vi "ep_Frequency Time Aggregation.vi"(0 "frequency (1/2) (half cycle)":dbl, 1 "restart (F)":bool, 5 "aggregation settings":T1={"interval"=1, "interval unit"=enum."Runs", "synchronization of intervals"=enum."Not synchronized", "algorithm"=enum."Average"}, 7 "voltage flags":bool[](array[boolean]), 9 "data time stamp":timestamp, 11 "error in (no error)":errorcluster) -> (6 "aggregated frequency":dbl, 8 "aggregated voltage flags":bool[](array[boolean]), 13 "aggregated data time stamp":timestamp, 14 "aggregated data valid?":bool, 15 "error out":errorcluster)   [LabVIEW 2011, in "NI_EP_Power Quality.lvlib"]
doc: "This VI accumulates input data. At every end of specified aggregation interval a minimum value, maximum value and average or RMS found within aggregation interval are provided on output. After this, the accumulation buffers are cleared and accumulation is automatically restarted."
uses:
  <vilib>/addons/Electrical Power/PQ/NI_EP_Power Quality.lvlib
  <vilib>/addons/Electrical Power/PQ/Common/Controls/ep_Aggregation Settings.ctl
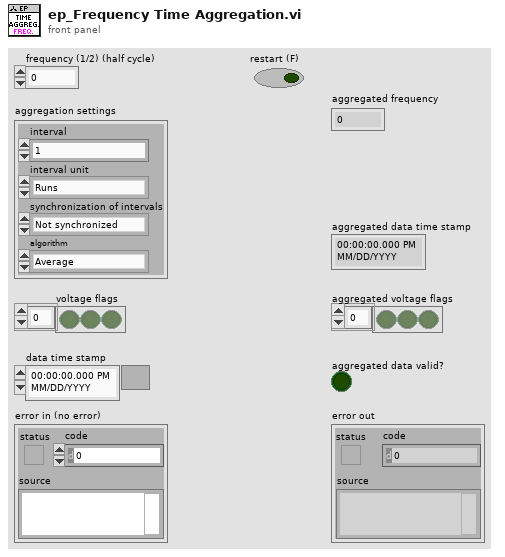
[diagram p1: front panel]
types:
  T1 = typedef "NI_EP_Power Quality.lvlib/ep_Aggregation Settings.ctl" = cluster{"interval":u32, "interval unit":enum16{"Runs", "Seconds", "Minutes", "Hours", "Days", "Weeks"}, "synchronization of intervals":enum16{"Not synchronized", "Interval rounded"}, "algorithm":enum16{"Average", "RMS"}}
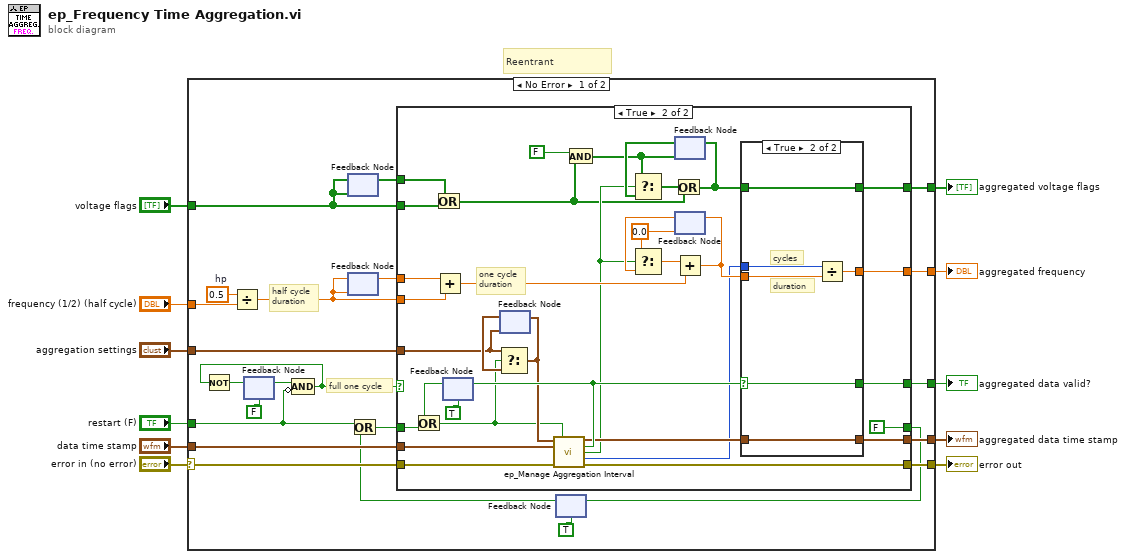
[diagram p0: block diagram]
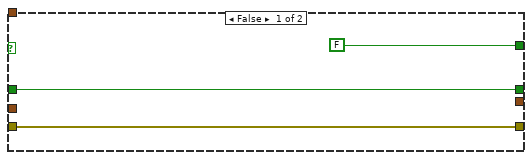
[diagram p2: hidden frame]
diagram:
  # "Reentrant"
  n1 = case shown="No Error" "error in (no error)" {
    selector: "error in (no error)" -> [w30 w79]
    tunnel: "restart (F)" -> [w19 _]
    tunnel: "frequency (1/2) (half cycle)" -> [w16 _]
    tunnel: "aggregation settings" -> [w28 _]
    tunnel: "data time stamp" -> [w34 _]
    tunnel: [w33 w79] -> w8
    tunnel: [w29 _] -> w7
    tunnel: [w32 _] -> w6
    tunnel: [w31 _] -> w5
    tunnel: "voltage flags" -> [w13 _]
    tunnel: [w14 _] -> w1
    frame No Error {
      w17 = 0.5  # hp
      # "half cycle\nduration"
      # "full one cycle"
      n2 = Divide(x=w17, y=w16) -> (x/y=w15:dbl)
      n3 = feedback #1(FALSE) -> (w27:bool)
      n4 = Compound Arithmetic op=AND(w27, invert w19) -> (w24:bool)
      n5 = Not(x=w24) -> (.not. x?=w26:bool)
      n6 = feedback-in #1(w26) -> ()
      n7 = feedback-in #2(w13) -> ()
      n8 = feedback #2(w13) -> (w12:bool[])
      n9 = feedback-in #3(w15) -> ()
      n10 = feedback #3(w15) -> (w23:dbl)
      n11 = feedback #4(TRUE) -> (w20:bool)
      n12 = Or(x=w19, y=w20) -> (x .or. y?=w18:bool)
      n13 = case shown="True" w24 {
        tunnel: w34 -> [_ w67]
        tunnel: [w36 w66] -> w33
        tunnel: [_ w64] -> w32
        tunnel: [_ w62] -> w31
        tunnel: w30 -> [w36 w61]
        tunnel: [FALSE w60] -> w29
        tunnel: w28 -> [_ w58]
        tunnel: w15 -> [_ w49]
        tunnel: w18 -> [w35 w53]
        tunnel: w23 -> [_ w50]
        tunnel: [w35 FALSE ("restart (F)")] -> w21
        tunnel: w13 -> [_ w39]
        tunnel: [_ w43] -> w14
        tunnel: w12 -> [_ w40]
        frame False {
        }
        frame True {
          w71 = 0.0
          # "one cycle\nduration"
          n14 = Or(x=w40, y=w39) -> (x .or. y?=w38:bool[])
          n15 = Add(x=w50, y=w49) -> (x+y=w52:dbl)
          n16 = feedback #5(TRUE) -> (w68:bool)
          n17 = Or(x=w68, y=w53) -> (x .or. y?=w42:bool)
          n18 = feedback #6(w58) -> (w59:T1)
          n19 = Select(t=w58, s=w42, f=w59) -> (s? t:f=w57:T1)
          n20 = feedback-in #6(w57) -> ()
          n21 = call <vilib>:"ep_Manage Aggregation Interval.vi"("aggregation settings"=w57, "restart (F)"=w42, "data time stamp"=w67, "error in (no error)"=w61) -> ("aggregated data time stamp"=w63:timestamp, "aggregated data valid?"=w65:bool, "restart aggregation?"=w41:bool, "runs"=w54:u32, "error out"=w66:errorcluster)  [unwired: 7 in]
          n22 = feedback-in #5(w65) -> ()
          n23 = And(x=FALSE, y=w38) -> (x .and. y?=w47:bool[])
          n24 = feedback #7(w47) -> (w48:bool[])
          n25 = Select(t=w47, s=w41, f=w48) -> (s? t:f=w46:bool[])
          n26 = Or(x=w46, y=w38) -> (x .or. y?=w44:bool[])
          n27 = feedback-in #7(w44) -> ()
          n28 = feedback #8(w71) -> (w70:dbl)
          n29 = Select(t=w71, s=w41, f=w70) -> (s? t:f=w56:dbl)
          n30 = Add(x=w56, y=w52) -> (x+y=w55:dbl)
          n31 = feedback-in #8(w55) -> ()
          n32 = case shown="True" w65 {
            selector: w65 -> [w72 w77]
            tunnel: [_ w75] -> w64
            tunnel: w55 -> [_ w76]
            tunnel: w63 -> [_ w78]
            tunnel: [_ w78] -> w62
            tunnel: [w72 w77] -> w60
            tunnel: w54 -> [_ w74]
            tunnel: [_ w73] -> w43
            tunnel: w44 -> [_ w73]
            frame False {
            }
            frame True {
              # "duration"
              # "cycles"
              n33 = Divide(x=w74, y=w76) -> (x/y=w75:dbl)
            }
          }
        }
      }
      n34 = feedback-in #4(w21) -> ()
    }
    frame Error {
    }
  }
  "error out" <- w8
  "aggregated frequency" <- w6
  "aggregated data valid?" <- w7
  "aggregated data time stamp" <- w5
  "aggregated voltage flags" <- w1
